vi "Connect to Slave.vi"(8 "error in (no error)":errorcluster, 11 "TCP master in":refnum<class "TCP Master.lvclass">) -> (0 "error out":errorcluster, 3 "TCP master out":refnum<class "TCP Master.lvclass">)   [LabVIEW 2021, in "TCP Master.lvclass"]
doc: "Opens a TCP connection to the address and port stored in the class."
uses:
  TCP Master.lvclass
  D:/my_projects/projects/Algorithms/Labview/21/Modbus_v121c/Network Protocol/Network Protocol.lvclass
  Network Protocol.lvclass/Network Protocol.ctl
  Transmission Data Unit/Transmission Data Unit.lvclass
  Network Protocol.lvclass
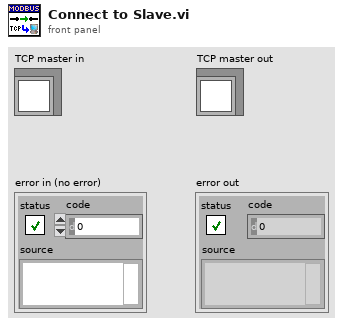
[diagram p1: front panel]
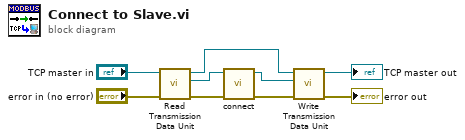
[diagram p0: block diagram]
diagram:
  n1 = call "Read Transmission Data Unit.vi"("error in (no error)"="error in (no error)", "Network Protocol in"="TCP master in") -> ("error out"=w4:errorcluster, "Transmission Data Unit"=w3:refnum<class "Transmission Data Unit.lvclass">, "Network Protocol out"=w9:refnum<class "TCP Master.lvclass">)  [unwired: 7 in]
  n2 = call-dynamic "connect.vi"("error in"=w4, "transmission data unit in"=w3) -> ("error out"=w2:errorcluster, "transmission data unit out"=w1:refnum<class "Transmission Data Unit.lvclass">)  [unwired: 8 in]
  n3 = call "Write Transmission Data Unit.vi"("error in (no error)"=w2, "Transmission Data Unit"=w1, "Network Protocol in"=w9) -> ("error out"=→"error out":errorcluster, "Network Protocol out"=→"TCP master out":refnum<class "TCP Master.lvclass">)  [unwired: 7 in]
